vi "Get Parameter.vi"(8 "error in (no error)":errorcluster, 11 "SolarSystems M266 Old in":refnum<class "SolarSystems M266 Old.lvclass">) -> (0 "error out":errorcluster, 2 "Parameter":refnum<class "AbstractData.lvclass">, 3 "SolarSystems M266 Old out":refnum<class "SolarSystems M266 Old.lvclass">)   [LabVIEW 2014, in "SolarSystems M266 Old.lvclass"]
uses:
  SolarSystems M266 Old.lvclass
  Framework/Model/Data/DataSingleElement/DataSingleElement.lvclass
  Framework/Model/Data/AbstractData/AbstractData.lvclass
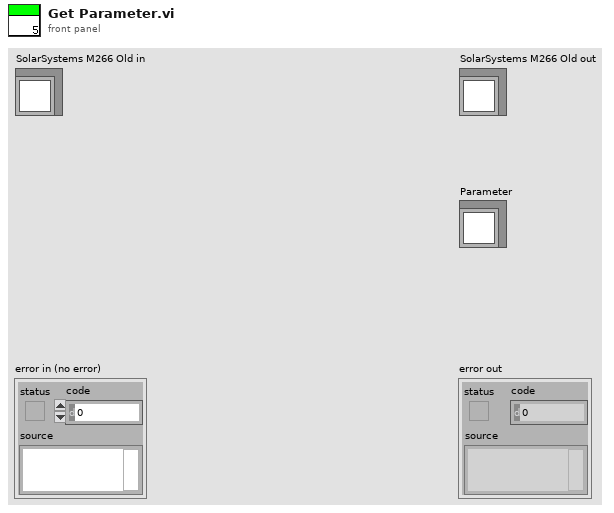
[diagram p1: front panel]
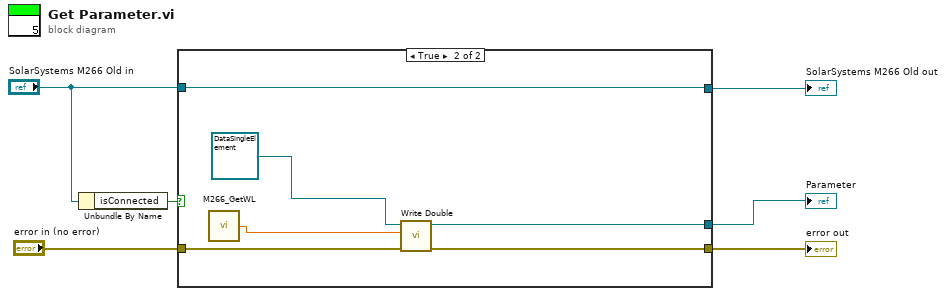
[diagram p0: block diagram]
diagram:
  n1 = Unbundle By Name("SolarSystems M266 Old in") -> ("isConnected"=w6:bool)
  n2 = case shown="True" w6 {
    tunnel: [w7 w11] -> w3
    tunnel: "error in (no error)" -> [w7 w12]
    tunnel: [w8 w14] -> w1
    tunnel: "SolarSystems M266 Old in" -> [w8 w14]
    tunnel: [_ w13] -> w2
    frame False {
    }
    frame True {
      n3 = call "M266_GetWL.vi"() -> ("Current WL"=w9:dbl)
      n4 = call "Write Double.vi"("error in (no error)"=w12, "value"=w9, "DataSingleElement in"=refnum<class "DataSingleElement.lvclass"> refnum ("DataSingleElement.lvclass")) -> ("error out"=w11:errorcluster, "DataSingleElement out"=w13:refnum<class "DataSingleElement.lvclass">)  [unwired: 7 in]
    }
  }
  "error out" <- w3
  "SolarSystems M266 Old out" <- w1
  "Parameter" <- w2
